vi "Delete Row.vi"(8 "error in (no error)":errorcluster, 10 "Row to Delete":i32, 11 "Ref In":refnum<vi>) -> (0 "error out":errorcluster)   [LabVIEW 2010]
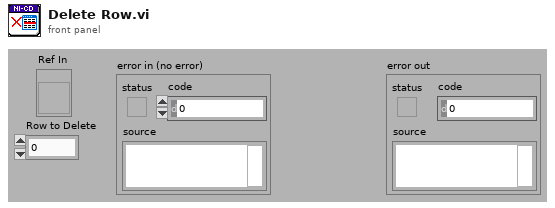
[diagram p1: front panel]
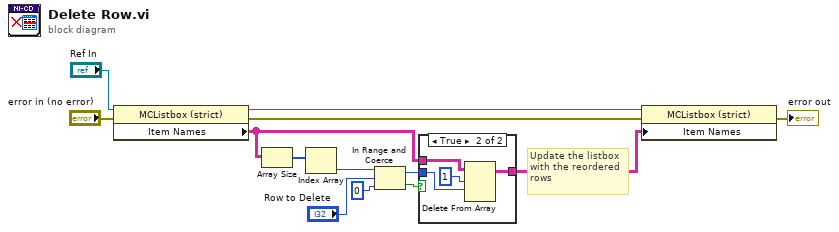
[diagram p0: block diagram]
diagram:
  # "Update the listbox\nwith the reordered\nrows"
  n1 = property class="MCListbox (strict)"(reference="Ref In", error in="error in (no error)") -> (reference out=w8:refnum<vi>, error out=w9:errorcluster, "Item Names"=w7:string[][])
  n2 = Array Size(array=w7) -> (size(s)=w6:i32[])
  n3 = Index Array(array=w6) -> (element=w4:i32)  [unwired: 1 in]
  n4 = In Range and Coerce(upper limit=w4, x="Row to Delete", lower limit=0) -> (coerced(x)=w2:i32, In Range?=w1:bool)
  n5 = case shown="True" w1 {
    tunnel: w7 -> [w14 w18]
    tunnel: [w14 w17] -> w10
    tunnel: w2 -> [_ w15]
    frame False {
    }
    frame True {
      n6 = Delete From Array(array=w18, length=1, index (row)=w15) -> (array with subset deleted=w17:string[][])  [unwired: 1 in, 1 out]
    }
  }
  n7 = property class="MCListbox (strict)"(reference=w8, error in=w9, "Item Names"=w10) -> (error out=→"error out":errorcluster)  [unwired: 1 out]
